vi "FTW-Actor-Broker-GetAddress.vi"(0 "FTW Message Broker":refnum<class "FTW-Actor-Broker.lvclass">, 11 "error in":errorcluster) -> (4 "FTW Message Broker out":refnum<class "FTW-Actor-Broker.lvclass">, 6 "Address":refnum<class "FTW-Actor-Address.lvclass">, 15 "error out":errorcluster)   [LabVIEW 2012, in "FTW-Actor-Broker.lvclass"]
uses:
  FTW-Actor-Broker.lvclass
  Address/FTW-Actor-Address.lvclass
  FTW-Actor-Broker.lvclass/FTW-Actor-Broker.ctl
panel:
  # "Inputs"
  # "Outputs"
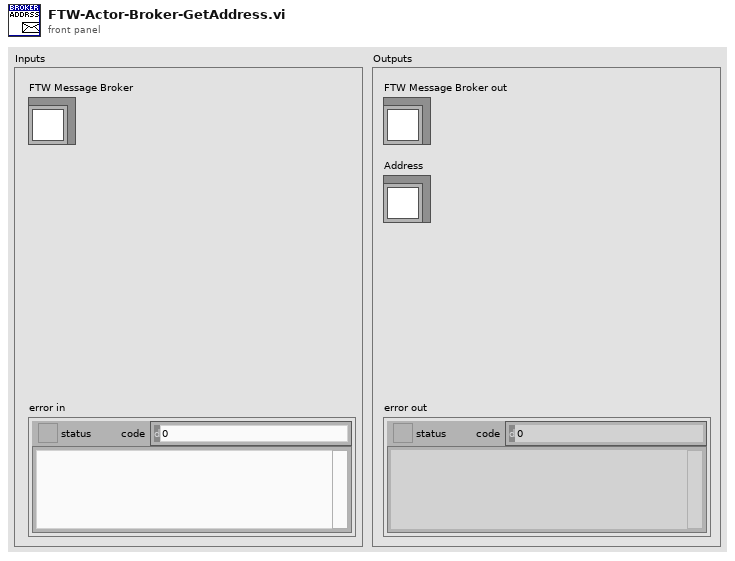
[diagram p1: front panel]
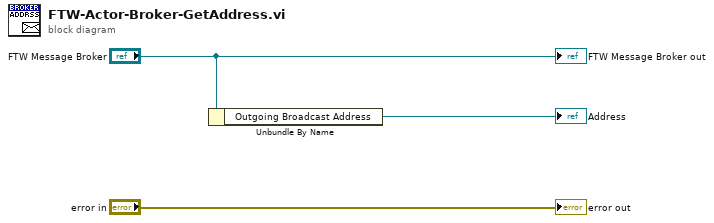
[diagram p0: block diagram]
diagram:
  n1 = Unbundle By Name("FTW Message Broker") -> ("Outgoing Broadcast Address"=→"Address":refnum<class "FTW-Actor-Address.lvclass">)
  "error out" <- "error in"
  "FTW Message Broker out" <- "FTW Message Broker"
